vi "SetExportType.vi"(8 "error in (no error)":errorcluster, 9 "Export type":T1, 11 "CGrapherDGML in":refnum<class "CGrapherDGML.lvclass">) -> (0 "error out":errorcluster, 3 "CGrapherDGML out":refnum<class "CGrapherDGML.lvclass">)   [LabVIEW 2020, in "DefaultExtensions.lvlib" / "CGrapherDGML.lvclass"]
uses:
  CGrapherDGML.lvclass
  ExtensionInterfaces/IExporter/ExportType.ctl
  CGrapherDGML.lvclass/CGrapherDGML.ctl
  ExtensionInterfaces/IExporter/IExporter.lvclass
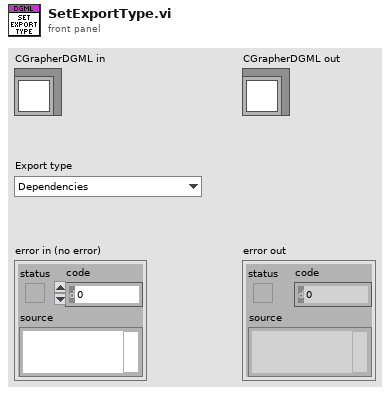
[diagram p1: front panel]
types:
  T1 = typedef "ExtensionInterfaces.lvlib/IExporter.lvclass/ExportType.ctl" = enum16{"Dependencies", "Rules", "Invalid dependencies", "Concessions", "Undeclared"}
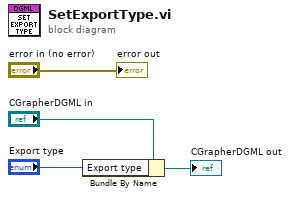
[diagram p0: block diagram]
diagram:
  n1 = Bundle By Name(cluster="CGrapherDGML in", "Export type"="Export type") -> (→"CGrapherDGML out":refnum<class "CGrapherDGML.lvclass">)
  "error out" <- "error in (no error)"
